vi "Turet Logic.vi"(6 "Turret Override?":bool, 7 "Manual Turret":dbl, 8 "Vision Target?":bool, 9 "Vision Xoffset":dbl, 10 "Shooting Position":T2, 11 "Driver Xoffset":dbl) -> (0 "Activate vision":bool, 1 "Turret Offset(degrees)":dbl, 2 "Turret mode":T1=enum."IMU", 3 "Scan Mode":bool)   [LabVIEW 2019, in "Robot.lvlib" / "Panzer.lvclass"]
uses:
  Panzer.lvclass
  PowerCellHandler/Controls/Shooting Position.ctl
  PowerCellHandler/Power Cell Handler.lvclass
  Turret/Controls/Turret control states.ctl
  Turret/Turret.lvclass
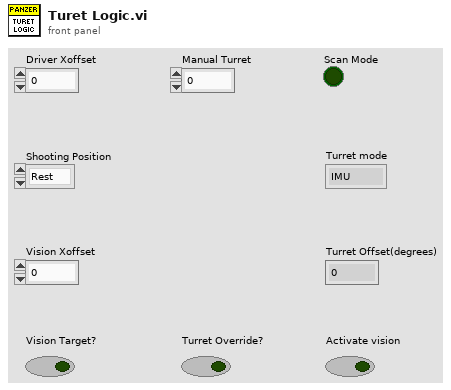
[diagram p1: front panel]
types:
  T1 = typedef "Turret.lvlib/Turret.lvclass/Turret control states.ctl" = enum16{"Position", "Offset", "IMU"}
  T2 = typedef "Power Cell Handler.lvlib/Power Cell Handler.lvclass/Shooting Position.ctl" = enum16{"Rest", "Front", "Middle", "Back"}
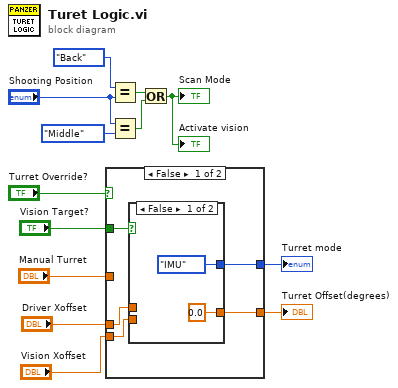
[diagram p0: block diagram]
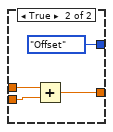
[diagram p2: hidden frame]
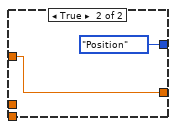
[diagram p3: hidden frame]
diagram:
  n1 = case shown="False" "Turret Override?" {
    tunnel: [w18 Turret_control_states."Position" ("Turret mode")] -> w7
    tunnel: [w17 w25] -> w6
    tunnel: "Driver Xoffset" -> [w16 _]
    tunnel: "Vision Xoffset" -> [w15 _]
    tunnel: "Vision Target?" -> [w14 _]
    tunnel: "Manual Turret" -> [_ w25]
    frame False {
      n2 = case shown="False" w14 {
        tunnel: [0.0 ("f") w21] -> w17
        tunnel: w15 -> [_ w22]
        tunnel: [Turret_control_states."IMU" ("Turret mode") Turret_control_states."Offset" ("Turret mode")] -> w18
        tunnel: w16 -> [_ w23]
        frame False {
        }
        frame True {
          n3 = Add(x=w23, y=w22) -> (x+y=w21:dbl)
        }
      }
    }
    frame True {
    }
  }
  "Turret mode" <- w7
  "Turret Offset(degrees)" <- w6
  n4 = Equal?(x=Shooting_Position."Back" ("Shooting Position"), y="Shooting Position") -> (x = y?=w10:bool)
  n5 = Equal?(x="Shooting Position", y=Shooting_Position."Middle" ("Shooting Position")) -> (x = y?=w9:bool)
  n6 = Or(x=w10, y=w9) -> (x .or. y?=→"Activate vision" →"Scan Mode":bool)
